vi "Read Owner GUID.vi"(8 "error in (no error)":errorcluster, 11 "Dependency in":refnum<class "Dependency.lvclass">) -> (0 "error out":errorcluster, 2 "Owner GUID":string, 3 "Dependency out":refnum<class "Dependency.lvclass">)   [LabVIEW 2021, in "smo.lvlib" / "Dependency.lvclass"]
uses:
  Dependency.lvclass
  Dependency.lvclass/Dependency.ctl
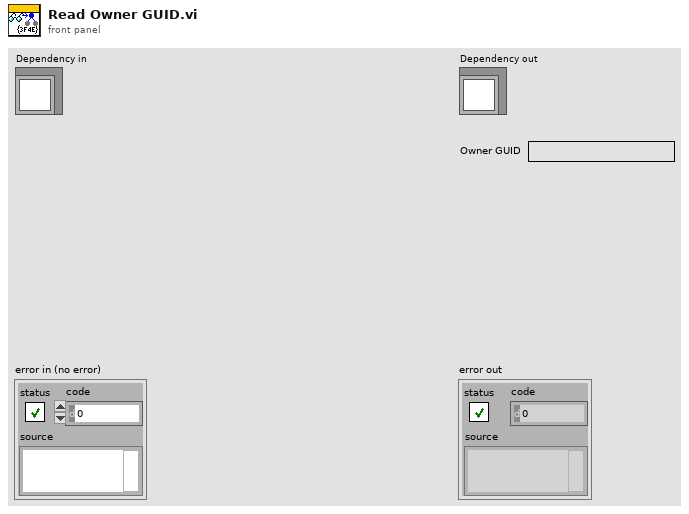
[diagram p1: front panel]
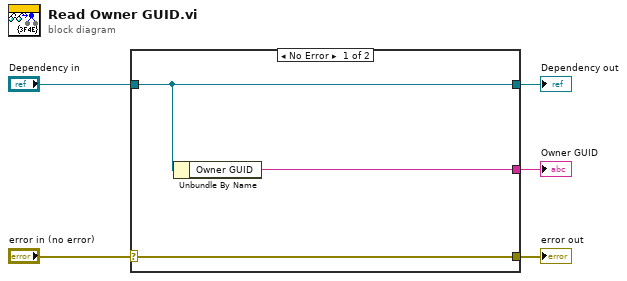
[diagram p0: block diagram]
diagram:
  n1 = case shown="No Error" "error in (no error)" {
    selector: "error in (no error)" -> [w8 w9]
    tunnel: [w8 w9] -> w4
    tunnel: [w7 w10] -> w2
    tunnel: "Dependency in" -> [w7 w10]
    tunnel: [w6 _] -> w1
    frame No Error {
      n2 = Unbundle By Name(w7) -> ("Owner GUID"=w6:string)
    }
    frame Error {
    }
  }
  "error out" <- w4
  "Dependency out" <- w2
  "Owner GUID" <- w1
